vi "Event Msg.vi"(10 "Event":refnum<data-value>) -> (0 "error out":errorcluster, 2 "Event Msg Strategy":refnum<user-event>)   [LabVIEW 2021, in "jettl.lvlib"]
uses:
  jettl.lvlib
  Msg Strategy/Msg Strategy/Msg Strategy.lvclass
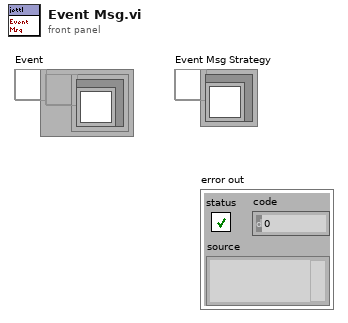
[diagram p1: front panel]
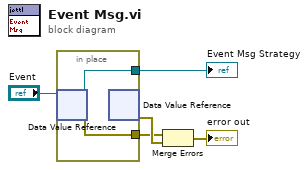
[diagram p0: block diagram]
diagram:
  n1 = in-place {
    in-place-border: [w7] -> w4
    in-place-border: [w6] -> w3
    n2 = in-place-dvr #1("Event") -> (w6:refnum<user-event>, w7:errorcluster)
    n3 = in-place-dvr #1() -> (w5:errorcluster)  [unwired: 1 in, 1 out]
  }
  "Event Msg Strategy" <- w3
  n4 = Merge Errors(w4, w5) -> (→"error out":errorcluster)
